vi "Pattern Classification.vi"() -> ()   [LabVIEW 2011, in "Super Simple Neural Network.lvlib"]
uses:
  Super Simple Neural Network.lvlib
  Types/Error Evaluation.ctl
  Types/Stop Settings.ctl
panel:
  in  "Stop Button":bool
  out "Response":bool[](array[boolean])=[FALSE, FALSE, FALSE, FALSE, FALSE, FALSE, FALSE, TRUE, FALSE, FALSE]
  in  "Pixels Pattern (play with this)":bool[][](array[boolean])=[[FALSE, FALSE, TRUE, TRUE, TRUE, FALSE, FALSE], [FALSE, TRUE, FALSE, FALSE, FALSE, TRUE, FALSE], [FALSE, TRUE, FALSE, FALSE, FALSE, TRUE, FALSE], [FALSE, TRUE, FALSE, FALSE, TRUE, FALSE, FALSE], [FALSE, FALSE, TRUE, TRUE, TRUE, FALSE, FALSE], [FALSE, TRUE, TRUE, FALSE, TRUE, TRUE, FALSE], [FALSE, TRUE, FALSE, FALSE, FALSE, TRUE, FALSE], [FALSE, TRUE, FALSE, FALSE, FALSE, TRUE, FALSE], [FALSE, TRUE, TRUE, TRUE, TRUE, TRUE, FALSE]]
  out "Error Trend":dbl[](graph)=[24.480125134800684, 16.67606596908778, 14.450878509911316, 12.59561764642866, 10.243351161394934, 10.348984586889003, 10.17078279361057, 10.097483515451659, 11.266914091147788, 10.996954328452704, 10.893596713204449, 10.230079417173886, 9.091616250608265, 8.856081147881168, 8.875285427642659, 8.899487792223038, 8.668389541585034, 8.534366472244649, 8.077293635966145, 8.009239857500013, 8.267824429010446, 8.02975984125342, 7.912837560396522, 7.837016648501839, 7.663473162515303, 7.315519801315367, 7.348481713006044, 7.261580792165606, 7.220142766544171, 7.0756624269432535, 6.776134882224065, 6.599572437966408, 6.431482700767773, 6.219595173353873, 6.216002379714119, 6.063679427720371, 5.965671920236437, 5.756656637158368, 5.637816651819244, 5.449511329779632, 5.329131928791041, 5.286399695194323, 5.21775274892969, 5.130142125103103, 5.093927694279854, 4.999495103500167, 4.849938977084474, 4.847309479398461, 4.61625975010939, 4.569836115790361, 4.503485570103185, 4.477428657702778, 4.344028397428328, 4.2238747285359715, 4.1087019792226, 4.030016036645038, 3.9989179442164606, 3.8591505403738977, 3.7866435633699673, 3.7585881764347544, 3.6451683755421715, 3.569440822258056, 3.4756540432889205, 3.4137126399231583, 3.358998701580505, 3.2809056315297656, 3.251185302779863, 3.1758957612606635, 3.1054583784755287, 3.0559907688750534, 3.050079931772938, 3.0284101810115174, 3.000863304993644, 2.9602897806747097, 2.9187516702076644, 2.8537697925798877, 2.825615398806235, 2.7890300938894477, 2.7751912840152575, 2.746432361451836, 2.7113339736314668, 2.6987698860587894, 2.647326852654893, 2.6201972174949253, 2.6142118782112327, 2.5787756888901994, 2.5546534176554756, 2.528863536434259, 2.4949248824612726, 2.451311122777462, 2.4363325318105176, 2.3985057951039663, 2.3654427859218026, 2.3408754184519234, 2.3370896729081823, 2.3062023682935364, 2.269247480752141, 2.274793297224241, 2.2736265612186006, 2.2573598692321424, 2.2332919642289246, 2.210594153250433, 2.1958429982216847, 2.167760306704811, 2.153603173422905, 2.1271651943266305, 2.1178735116998757, 2.1094446764766106, 2.0986643415917468, 2.08640254230974, 2.1111684892724476, 2.1021103297182684, 2.0829157561541396, 2.0757034760397275, 2.076459619542023, 2.072875633456028, 2.045290527344823, 2.045166124939432, 2.0120529010196737, 2.007515495355189, 1.99541472258216, 1.9731228435434365, 1.9530408084864823, 1.9401759513290218, 1.931838755920019, 1.9244373593540494, 1.9179433500293386, 1.9116672212550323, 1.9011342312630357, 1.8859339403959448, 1.8714116235385705, 1.8550061671747287, 1.8431089338137139, 1.8281511617333288, 1.8129949802606626, 1.8007790085885227, 1.777117965843751, 1.7641928479816584, 1.7636614831823247, 1.7453534497955598, 1.753219464031541, 1.7155553000449713, 1.7033528408077865, 1.7180280172635638, 1.7102534277264028, 1.689499347120349, 1.681134349380529, 1.6708368320412883, 1.6714826187088483, 1.6498682764689414, 1.6227280287117702, 1.6025888011911062, 1.588575711635777, 1.5736973486522492, 1.5629262118567262, 1.5370500884671132, 1.5274581187753729, 1.5160890598175012, 1.4777804575372229, 1.4928377405208393, 1.4757470089517917, 1.4609862551027102, 1.4659153193997583, 1.4421298209555145, 1.415044812556455, 1.4013377134559144, 1.4221394681397084, 1.4125527862609784, 1.397018126307822, 1.3926436427870978, 1.372651146595268, 1.3669006227702722, 1.3543263648122035, 1.339703825946739, 1.3307136541066868, 1.3284630425645443, 1.3299989944722799, 1.305876794322784, 1.2866999323394985, 1.285820748227145, 1.2828662906179835, 1.2781866844565524, 1.3120049457065928, 1.271549886758931, 1.2557287986605112, 1.2522955520819425, 1.2567096461385754, 1.2528717763680335, 1.243195002690183, 1.2282752947938715, 1.2219083564457733, 1.2254137360202515, 1.2179085174665714, 1.203304065599701, 1.1936118247411283, 1.2082344998530958, 1.2017585664777188, 1.1965418584180905, 1.189754563548206, 1.1868250139209715, 1.1949336696537347, 1.194584158237879, 1.1864302120050252, 1.191577447230282, 1.1899944135522, 1.1995127258606006, 1.1785864499557528, 1.1845462489347578, 1.182157585998869, 1.1652149293174467, 1.1595963087270258, 1.1603917067631127, 1.1573180107598455, 1.1561878541661708, 1.1406169067010887, 1.1316220683935867, 1.1283707254969118, 1.1141813887573389, 1.1098488603658936, 1.1219574221558353, 1.1003881256409982, 1.108911351615352, 1.1193494127796235, 1.1149606169108972, 1.117893413738126, 1.1177635253826153, 1.1128915372838313, 1.1087270173858943, 1.1100222103276152, 1.1050351258640183, 1.0958461724869346, 1.0932791878383215, 1.0917286141105014, 1.087256924313096, 1.0780002764523526, 1.0786506223865353, 1.0789302048894511, 1.0957882744879304, 1.057486592133635, 1.0788395237190147, 1.0746062381858033, 1.0504126173959893, 1.023326399965327, 1.0282002946276632, 1.0196214969263064, 1.0100498192138723, 0.9911932894406601]
  # "1"
  # "2"
  # "3"
  # "4"
  # "5"
  # "6"
  # "7"
  # "8"
  # "9"
  # "0"
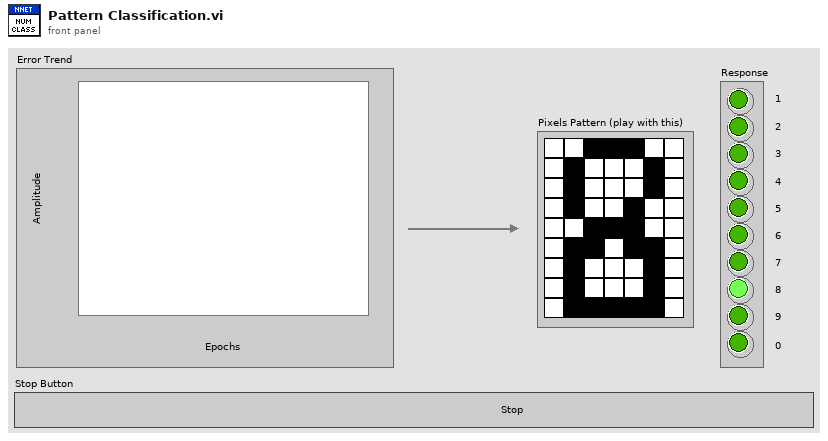
[diagram p1: front panel]
types:
  T1 = typedef "Super Simple Neural Network.lvlib/Stop Settings.ctl" = cluster{"Max Epocs":u64, "Error Goal":dbl, "Max Time (s)":dbl, "Error Evaluation":T2}
  T2 = typedef "Super Simple Neural Network.lvlib/Error Evaluation.ctl" = enum16{"Over Both Sets", "Over Validation Set", "Over Teaching Set"}
  T3 = typedef "Super Simple Neural Network.lvlib/Neural Network.ctl" = cluster{"Weigths":T4[], "Last Layer Linear":bool, "Add Bias Inputs":bool, "# Inputs":u32, "# Output Neurons/Outputs":u32, "Inputs Scaling":T5, "Outputs Scaling":T5}
  T4 = typedef "Super Simple Neural Network.lvlib/2D Array.ctl" = cluster{"2D Array":dbl[][]}
  T5 = typedef "Super Simple Neural Network.lvlib/Scaling Info.ctl" = cluster{"X Scaling Vector":dbl[], "Y Scaling Vector":dbl[]}
  T6 = typedef "Super Simple Neural Network.lvlib/Teaching Vector.ctl" = cluster{"Inputs":T7, "Expected Outputs":T7}
  T7 = typedef "Super Simple Neural Network.lvlib/1D Array.ctl" = cluster{"1D Array":dbl[]}
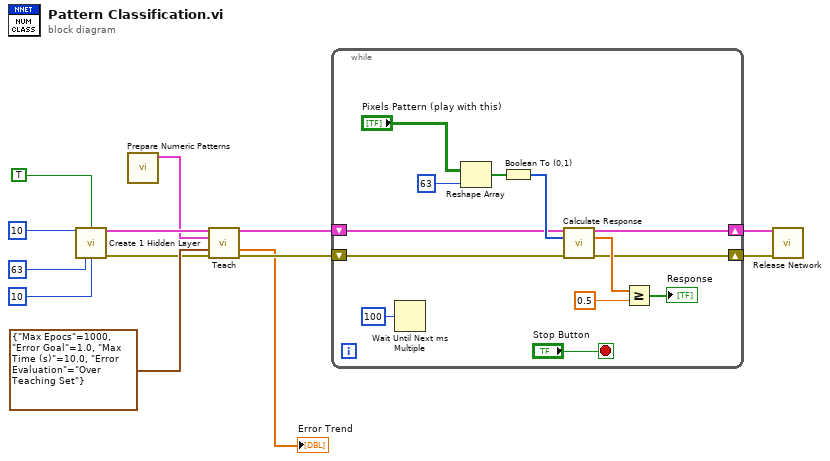
[diagram p0: block diagram]
diagram:
  n1 = call "Create 1 Hidden Layer.vi"("1st Hidden Layer Neurons"=u32 10, "Add Bias Inputs"=TRUE, "# Inputs"=u32 63, "Output Neurons/Outputs"=u32 10) -> ("Neural Network Out"=w13:T3, "Error Out"=w6:errorcluster)  [unwired: 10 in]
  n2 = call "Prepare Numeric Patterns.vi"() -> ("Numeric Patterns"=w8:T6[])  [unwired: 11 in]
  n3 = call "Teach.vi"("Neural Network In"=w13, "Teaching Set In"=w8, "Termination Settings In"=T1 {"Max Epocs"=1000, "Error Goal"=1.0, "Max Time (s)"=10.0, "Error Evaluation"=enum."Over Teaching Set"}, "Error In"=w6) -> ("Neural Network Out"=w5:T3, "Error Trend Out"=→"Error Trend":dbl[], "Error Out"=w4:errorcluster)  [unwired: 8 in, 1 out]
  n4 = while {
    shift-right: [w17] -> w3
    shift-left: w5 -> [w19]
    shift-right: [w16] -> w2
    shift-left: w4 -> [w18]
    stop <- "Stop Button" stop-if-true
    n5 = Wait Until Next ms Multiple(millisecond multiple=u32 100) -> ()  [unwired: 1 out]
    n6 = Reshape Array("Pixels Pattern (play with this)", 63 ("dimension size")) -> (w26:bool[])
    n7 = Boolean To (0,1)(Boolean=w26) -> (0, 1=w23:i16[])
    n8 = call "Calculate Response.vi"("Neural Network In"=w19, "Inputs"=w23, "Error In"=w18) -> ("Neural Network Out"=w17:T3, "Outputs"=w22:dbl[], "Error Out"=w16:errorcluster)  [unwired: 10 in]
    n9 = Greater Or Equal?(x=w22, y=0.5) -> (x >= y?=→"Response":bool[])
  }
  n10 = call "Release Network.vi"("Neural Network"=w3, "Error In"=w2) -> ()  [unwired: 13 in, 1 out]
